vi "AngleCorrection.vi"(8 "error in (no error)":errorcluster, 11 "Numeric in":dbl) -> (0 "error out":errorcluster, 3 "Numeric out":dbl)   [LabVIEW 2019, in "Algorithm.lvclass"]
uses:
  FrameworkOverrides/Algorithm.lvclass
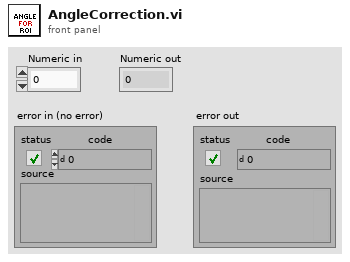
[diagram p1: front panel]
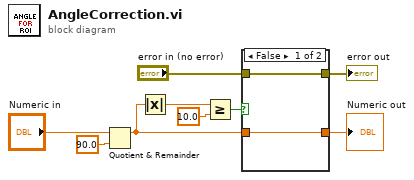
[diagram p0: block diagram]
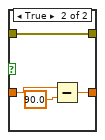
[diagram p2: hidden frame]
diagram:
  n1 = Quotient & Remainder(x="Numeric in", y=90.0) -> (x-y*floor(x/y)=w9:dbl)  [unwired: 1 out]
  n2 = Absolute Value(x=w9) -> (abs(x)=w7:dbl)
  n3 = Greater Or Equal?(x=w7, y=10.0) -> (x >= y?=w6:bool)
  n4 = case shown="False" w6 {
    tunnel: w9 -> [w11 w14]
    tunnel: [w11 w13] -> w5
    tunnel: "error in (no error)" -> [w10 w12]
    tunnel: [w10 w12] -> w1
    frame False {
    }
    frame True {
      n5 = Subtract(x=w14, y=90.0) -> (x-y=w13:dbl)
    }
  }
  "Numeric out" <- w5
  "error out" <- w1
